vi "entity set UEI16.vi"(0 "id":u32, 1 "option":i32, 2 "inValue":i32, 5 "result":cluster{"value":i32, "error":i32}, 7 "entity":i32, 9 "index":i32, 11 "error in (no error)":errorcluster, 12 "param":i32) -> (4 "id out":u32, 6 "result out":cluster{"value":i32, "error":i32}, 15 "error out":errorcluster)   [LabVIEW 2014, in "BrainStem2_LabVIEW_Library.lvlib"]
doc: "aLIBEXPORT void __stdcall entity_setUEI16(unsigned int* id, struct Result* result, int entity = 0, int index = 0, int option = 0, int param = -1, int inValue = 0);"
uses:
  BrainStem2_LabVIEW_Library.lvlib
  BrainStem2_LabVIEW.dll
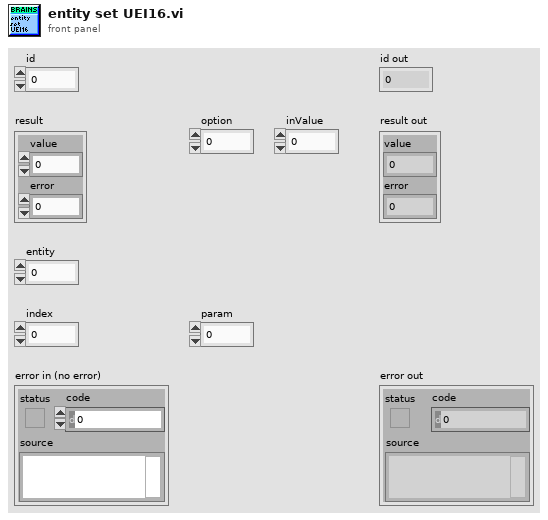
[diagram p1: front panel]
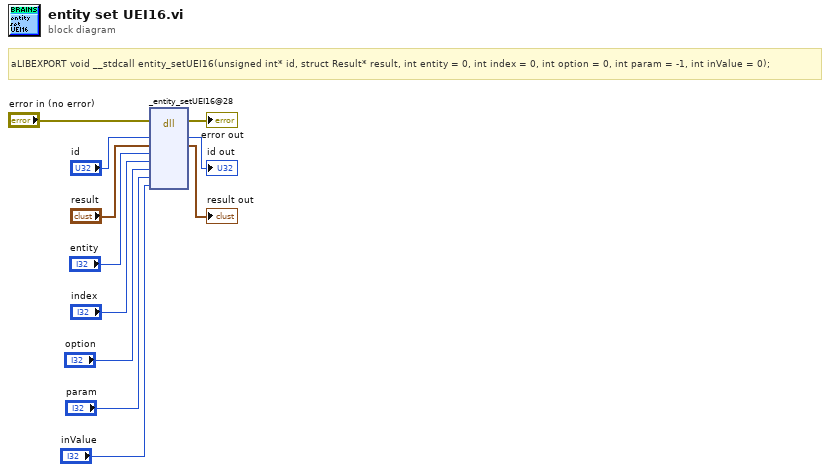
[diagram p0: block diagram]
diagram:
  # "aLIBEXPORT void __stdcall entity_setUEI16(unsigned int* id, struct Result* result, int entity = 0, int index = 0, int option = 0, int param = -1, int inValue = 0);"
  n1 = dll-call lib="C:/Users/mitch/Documents/development/acroname/software/acroname/aSource/BrainStem2/BrainStem2_LabVIEW/LabVIEW_2014_Distribution/BrainStem2_LabVIEW_w32/BrainStem2_LabVIEW.*" fn="_entity_setUEI16@28"(error in="error in (no error)", "id"="id", "result"="result", "entity"="entity", "index"="index", "option"="option", "param"="param", "inValue"="inValue") -> (error out=→"error out":errorcluster, "id"=→"id out":u32, "result"=→"result out":cluster{"value":i32, "error":i32})  [unwired: 8 in, 1 out]
